vi "CAN Jaguar Get Position Reference.vi"(8 "error in (no error)":errorcluster, 11 "CAN Jaguar Ref":T1={"Device Number"=0, "Control Mode"=enum."Percent VBus", "Inverted"=FALSE, "Semaphore"=refnum, "Max Vout"=12.0, "DevStatus"={"status"=FALSE, "code"=0, "source"=""}}) -> (0 "error out":errorcluster, 2 "Position Reference":T4, 3 "CAN Jaguar Ref Out":T1={"Device Number"=0, "Control Mode"=enum."Percent VBus", "Inverted"=FALSE, "Semaphore"=refnum, "Max Vout"=12.0, "DevStatus"={"status"=FALSE, "code"=0, "source"=""}})   [LabVIEW 2009, in "CAN.lvlib"]
uses:
  CAN.lvlib
  SubVIs/CAN Motor Message IDs.ctl
  SubVIs/CAN Jaguar Position Reference.ctl
  SubVIs/CAN Jaguar Control Mode.ctl
  SubVIs/CAN Jaguar Ref.ctl
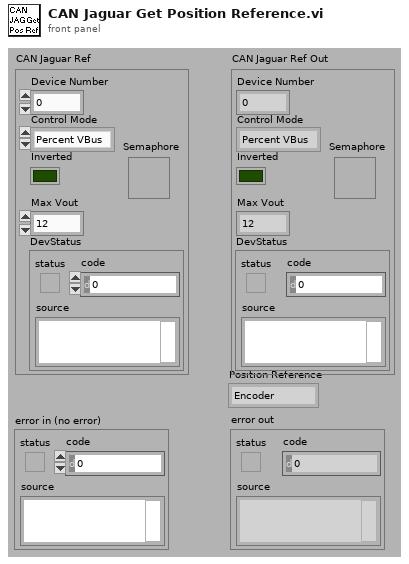
[diagram p1: front panel]
types:
  T1 = typedef "CAN.lvlib/CAN Jaguar Ref.ctl" = cluster{"Device Number":u8, "Control Mode":T2, "Inverted":bool, "Semaphore":T3, "Max Vout":dbl, "DevStatus":errorcluster}
  T2 = typedef "CAN.lvlib/CAN Jaguar Control Mode.ctl" = enum16{"Percent VBus", "Speed", "Position", "Current"}
  T3 = typedef "Semaphore RefNum" = refnum<k1>
  T4 = typedef "CAN.lvlib/CAN Jaguar Position Reference.ctl" = enum16{"Encoder", "Potentiometer"}
  T5 = enum16{"big-endian, network order", "native, host order", "little-endian"}
  T6 = typedef "CAN.lvlib/CAN Motor Message IDs.ctl" = u32
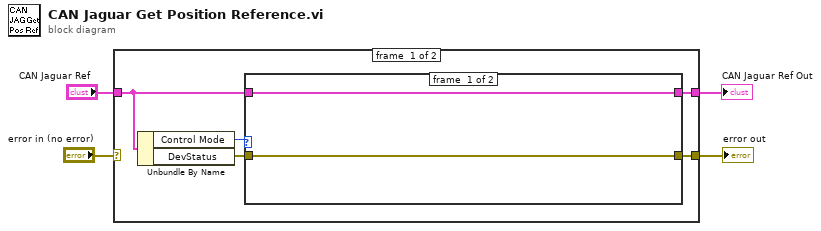
[diagram p0: block diagram]
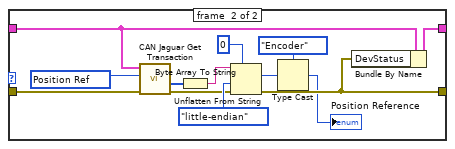
[diagram p2: hidden frame]
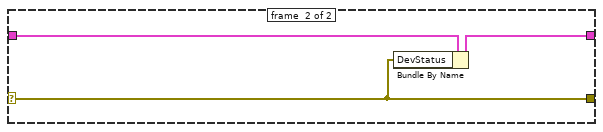
[diagram p3: hidden frame]
diagram:
  n1 = case shown="No Error" "error in (no error)" {
    selector: "error in (no error)" -> [_ w25]
    tunnel: [w5 w26] -> w4
    tunnel: "CAN Jaguar Ref" -> [w7 w27]
    tunnel: [w9 w25] -> w2
    frame #0 {
      n2 = Unbundle By Name(w7) -> ("Control Mode"=w8:T2, "DevStatus"=w6:errorcluster)
      n3 = case shown="\"Position\"" w8 {
        tunnel: [w11 w15] -> w9
        tunnel: w7 -> [w10 w14]
        tunnel: w6 -> [w11 w17]
        tunnel: [w10 w13] -> w5
        frame #0 {
        }
        frame #1 {
          w16 = T6 33688960 items=["Volt Enable"=33685504, "Volt Disable"=33685568, "Volt Set"=33685632, "Volt Set Ramp"=33685696, "Speed Enable"=33686528, "Speed Disable"=33686592, "Speed Set"=33686656, "Speed P"=33686720, "Speed I"=33686784, "Speed D"=33686848, "Speed Ref"=33686912, "Position Enable"=33688576, "Position Disable"=33688640, "Position Set"=33688704, "Position P"=33688768, "Position I"=33688832, "Position D"=33688896, "Position Ref"=33688960, "Current Enable"=33689600, "Current Disable"=33689664, "Current Set"=33689728, "Current P"=33689792, "Current I"=33689856, "Current D"=33689920, "Status VOut"=33690624, "Status VBus"=33690688, "Status Current"=33690752, "Status Temp"=33690816, "Status Position"=33690880, "Status Speed"=33690944, "Status Limit"=33691008, "Status Fault"=33691072, "Status Power"=33691136, "Config Num Brushes"=33692672, "Config Encoder Lines"=33692736, "Config Pot Turns"=33692800, "Config Brake Coast"=33692864, "Config Limit Mode"=33692928, "Config Limit Fwd"=33692992, "Config Limit Rev"=33693056, "Config Max VOut"=33693120, "Config Fault Time"=33693184, "Motor Ack"=33693696] ("CAN Motor Message IDs")
          n4 = call "CAN Jaguar Get Transaction.vi"("error in"=w17, "Message ID"=w16, "CAN Jaguar Ref"=w14) -> ("error out"=w19:errorcluster, "Data"=w18:u8[])  [unwired: 7 out]
          n5 = Byte Array To String(unsigned byte array=w18) -> (string=w23:string)
          n6 = Unflatten From String(type=u8 0 ("Voltage"), binary string=w23, byte order (0:big-endian, network order)=T5."little-endian", error in (no error)=w19) -> (value=w22:u8, error out=w15:errorcluster)  [unwired: 2 out]
          n7 = Type Cast(type=CAN_Jaguar_Position_Reference."Encoder" ("Position Reference"), x=w22) -> (*(type *) &x=→"Position Reference":T4)
          n8 = Bundle By Name(cluster=w14, "DevStatus"=w15) -> (w13:T1)
        }
      }
    }
    frame #1 {
      n9 = Bundle By Name(cluster=w27, "DevStatus"=w25) -> (w26:T1)
    }
  }
  "CAN Jaguar Ref Out" <- w4
  "error out" <- w2
